vi "HTTP GET.vi"(2 "error IO":errorcluster, 3 "URI":string) -> (0 "error out":errorcluster, 1 "body":string)   [LabVIEW 2012]
panel:
  out "Timed Out?":bool
  out "Returned Header":string
  out "concatenated string":string
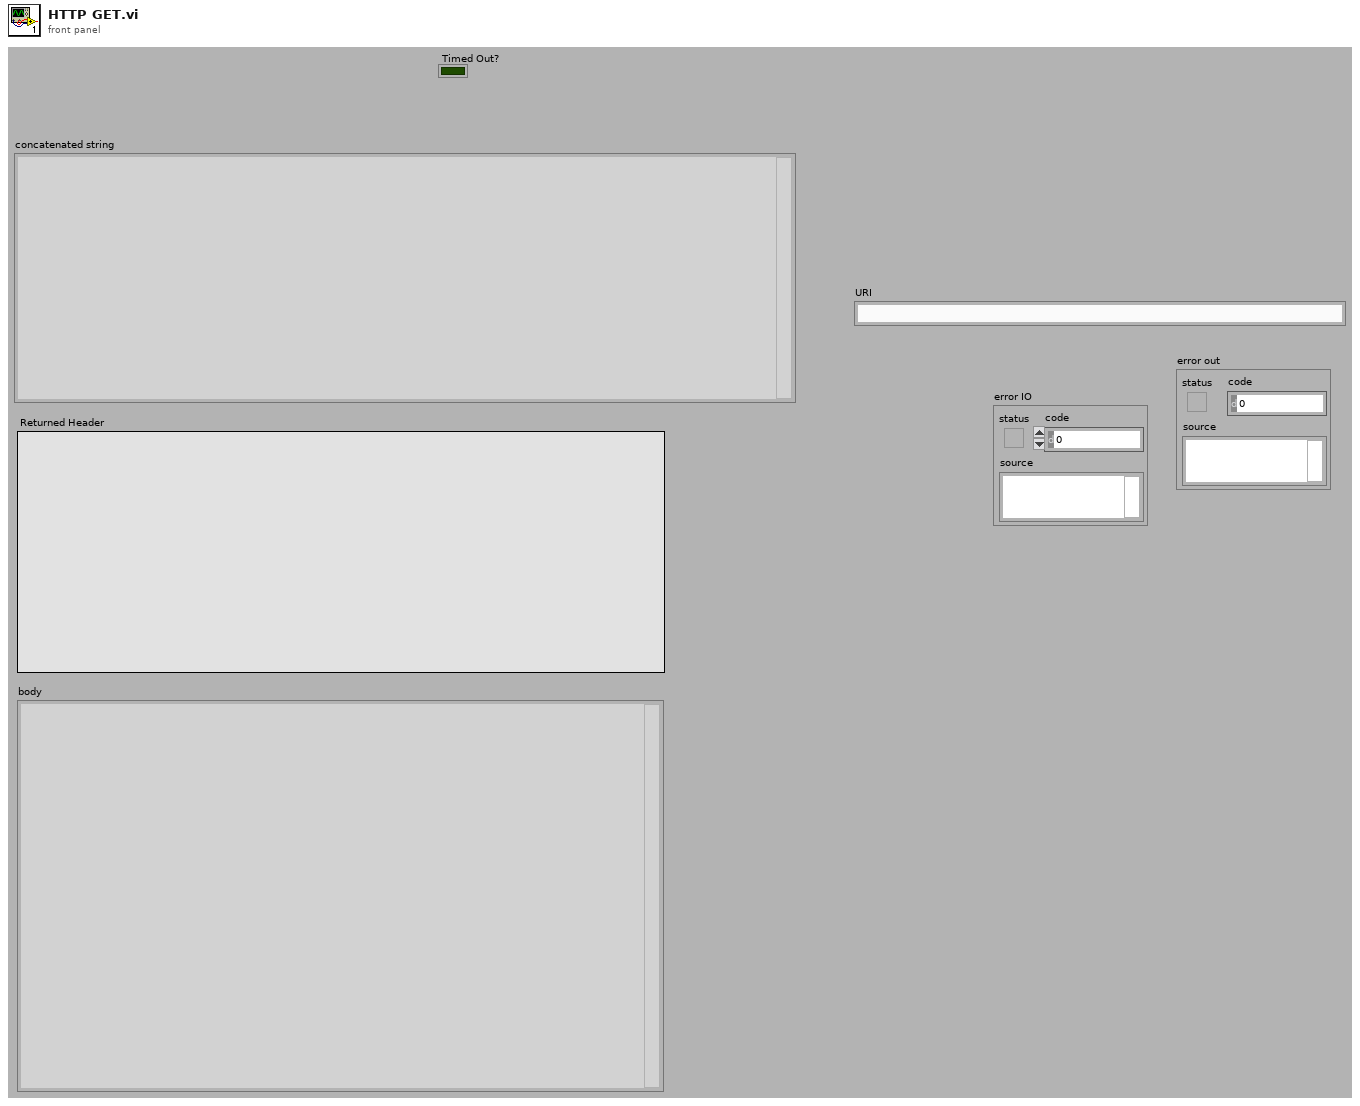
[diagram p1: front panel]
types:
  T1 = enum16{"Standard", "Buffered", "CRLF", "Immediate"}
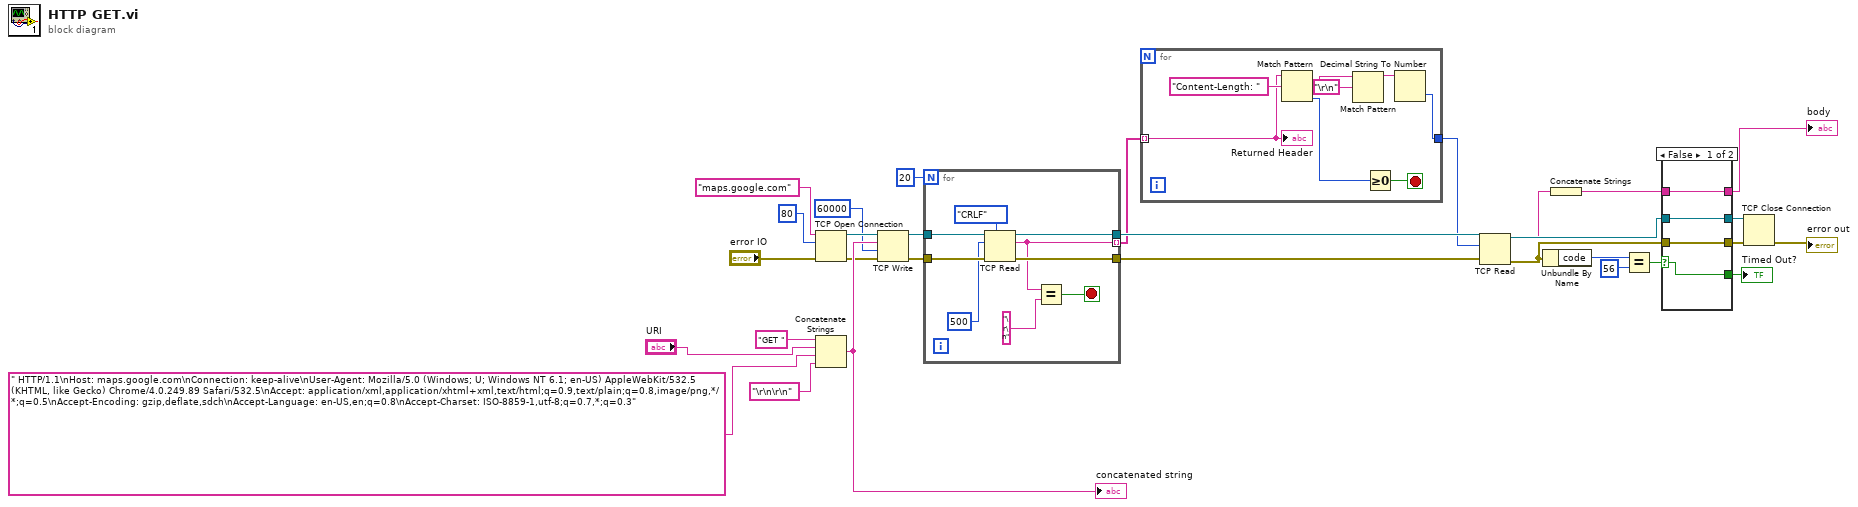
[diagram p0: block diagram]
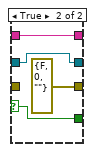
[diagram p2: hidden frame]
diagram:
  n1 = TCP Open Connection(address="maps.google.com", remote port or service name=u16 80 ("remote port"), error in (no error)="error IO") -> (connection ID=w18:refnum<k5>, error out=w17:errorcluster)  [unwired: 2 out]
  n2 = Concatenate Strings("GET " ("Command"), "URI", " HTTP/1.1\nHost: maps.google.com\nConnection: keep-alive\nUser-Agent: Mozilla/5.0 (Windows; U; Windows NT 6.1; en-US) AppleWebKit/532.5 (KHTML, like Gecko) Chrome/4.0.249.89 Safari/532.5\nAccept: application/xml,application/xhtml+xml,text/html;q=0.9,text/plain;q=0.8,image/png,*/*;q=0.5\nAccept-Encoding: gzip,deflate,sdch\nAccept-Language: en-US,en;q=0.8\nAccept-Charset: ISO-8859-1,utf-8;q=0.7,*;q=0.3" ("Command"), "\r\n\r\n" ("string")) -> (w19:string)
  "concatenated string" <- w19
  n3 = TCP Write(connection ID=w18, data in=w19, error in (no error)=w17, 9:60000 ("timeout ms (25000)")) -> (connection ID out=w15:refnum<k5>, error out=w14:errorcluster)  [unwired: 1 out]
  n4 = for {
    N: 20 -> [_]
    tunnel: w15 -> [w39]
    tunnel: w14 -> [w38]
    tunnel: [w37] -> w13
    tunnel: [w36] -> w12
    tunnel: [w33] -> w11 mode=indexing
    stop <- w32 stop-if-true
    n5 = TCP Read(connection ID=w39, bytes to read=500, error in (no error)=w38, 7:T1."CRLF" ("mode (standard)")) -> (connection ID out=w36:refnum<k5>, data out=w33:string, error out=w37:errorcluster)  [unwired: 1 in]
    n6 = Equal?(x=w33, y="\r\n" ("data out")) -> (x = y?=w32:bool)
  }
  n7 = for {
    tunnel: w11 -> [w44] mode=indexing
    tunnel: [w42] -> w10
    stop <- w41 stop-if-true
    n8 = Match Pattern(string=w44, regular expression="Content-Length: ") -> (after substring=w46:string, offset past match=w40:i32)  [unwired: 3 out]
    n9 = Match Pattern(string=w46, regular expression="\r\n") -> (before substring=w43:string)  [unwired: 4 out]
    n10 = Greater Or Equal To 0?(x=w40) -> (x >= 0?=w41:bool)
    n11 = Decimal String To Number(string=w43) -> (number=w42:i32)  [unwired: 3 out]
    "Returned Header" <- w44
  }
  n12 = TCP Read(connection ID=w12, bytes to read=w10, error in (no error)=w13) -> (connection ID out=w26:refnum<k5>, data out=w24:string, error out=w23:errorcluster)  [unwired: 1 in, 1 out]
  n13 = Unbundle By Name(w23) -> ("code"=w20:i32)
  n14 = Concatenate Strings(w24) -> (w25:string)
  n15 = Equal?(x=w20, y=56) -> (x = y?=w21:bool)
  n16 = case shown="False" w21 {
    selector: w21 -> [w48 w52]
    tunnel: [w49 w54] -> w4
    tunnel: w25 -> [w49 w54]
    tunnel: [w51 errorcluster {"status"=FALSE, "code"=0, "source"=""} ("error in (no error)")] -> w28
    tunnel: w23 -> [w51 _]
    tunnel: w26 -> [w50 w53]
    tunnel: [w50 w53] -> w27
    tunnel: [w48 w52] -> w8
    frame False {
    }
    frame True {
    }
  }
  "body" <- w4
  "Timed Out?" <- w8
  n17 = TCP Close Connection(connection ID=w27, error in (no error)=w28) -> (error out=→"error out":errorcluster)  [unwired: 2 out]
